vi "Write Subpanel Refnum.vi"(7 "Force Overwrite? (F)":bool, 8 "error in (no error)":errorcluster, 10 "SubPnl Refnum":refnum<vi>, 11 "IViewModel In":refnum<class "IViewModel.lvclass">) -> (0 "error out":errorcluster, 3 "IViewModel Out":refnum<class "IViewModel.lvclass">)   [LabVIEW 2015, in "IViewModel.lvlib" / "IViewModel.lvclass"]
doc: "<License>\nCopyright © 2017 Composed Systems, LLC | All rights reserved\nwww.composed.io\n\nAuthor: Ethan Stern <ethan.stern@composed.io>\n\nThis software is provided \"AS IS\" WITHOUT WARRANTIES, either express or implied, AND IS FOR EDUCATIONAL PURPOSES ONLY.\n</License>"
uses:
  IViewModel.lvclass
  IViewModel.lvclass/IViewModel.ctl
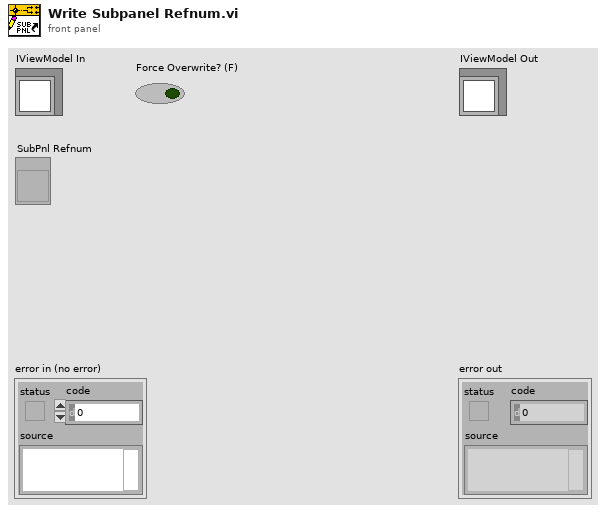
[diagram p1: front panel]
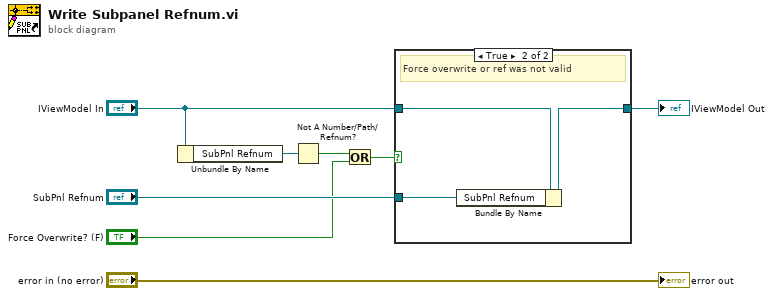
[diagram p0: block diagram]
diagram:
  n1 = Unbundle By Name("IViewModel In") -> ("SubPnl Refnum"=w5:refnum<vi>)
  n2 = Not A Number/Path/Refnum?(number/path/refnum=w5) -> (NaN/Path/Refnum?=w4:bool)
  n3 = Or(x=w4, y="Force Overwrite? (F)") -> (x .or. y?=w1:bool)
  n4 = case shown="True" w1 {
    tunnel: [w9 w12] -> w7
    tunnel: "SubPnl Refnum" -> [_ w11]
    tunnel: "IViewModel In" -> [w9 w10]
    frame False {
      # "Keep pre-existing refnum"
    }
    frame True {
      # "Force overwrite or ref was not valid"
      n5 = Bundle By Name(cluster=w10, "SubPnl Refnum"=w11) -> (w12:refnum<class "IViewModel.lvclass">)
    }
  }
  "IViewModel Out" <- w7
  "error out" <- "error in (no error)"
